vi "Day7Part2.vi"(11 "Input":string="190: 10 19\n3267: 81 40 27\n83: 17 5\n156: 15 6\n7290: 6 8 6 15\n161011: 16 10 13\n192: 17 8 14\n21037: 9 7 18 13\n292: 11 6 16 20") -> (3 "Result":u64)   [LabVIEW 2024]
uses:
  <vilib>/Utility/error.llb/Trim Whitespace One-Sided.vi
  <userlib>/_OpenG.lib/string/string.llb/openg_string.lvlib
panel:
  out "Answers":u64[](array[numeric])
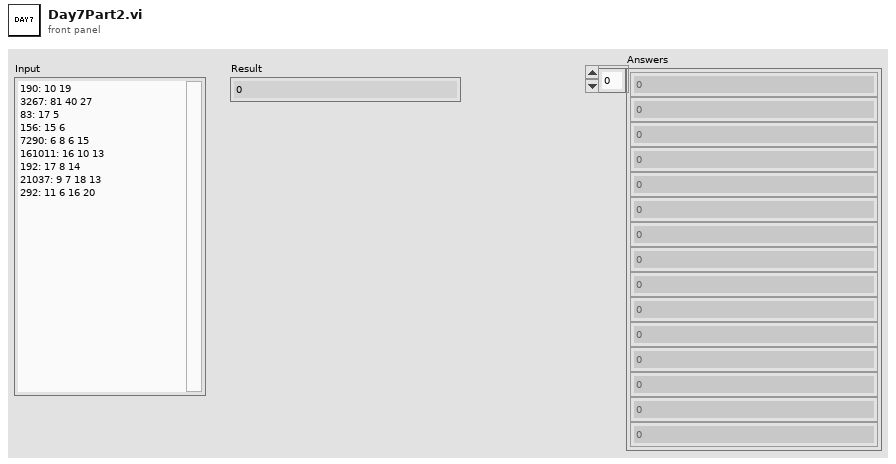
[diagram p1: front panel]
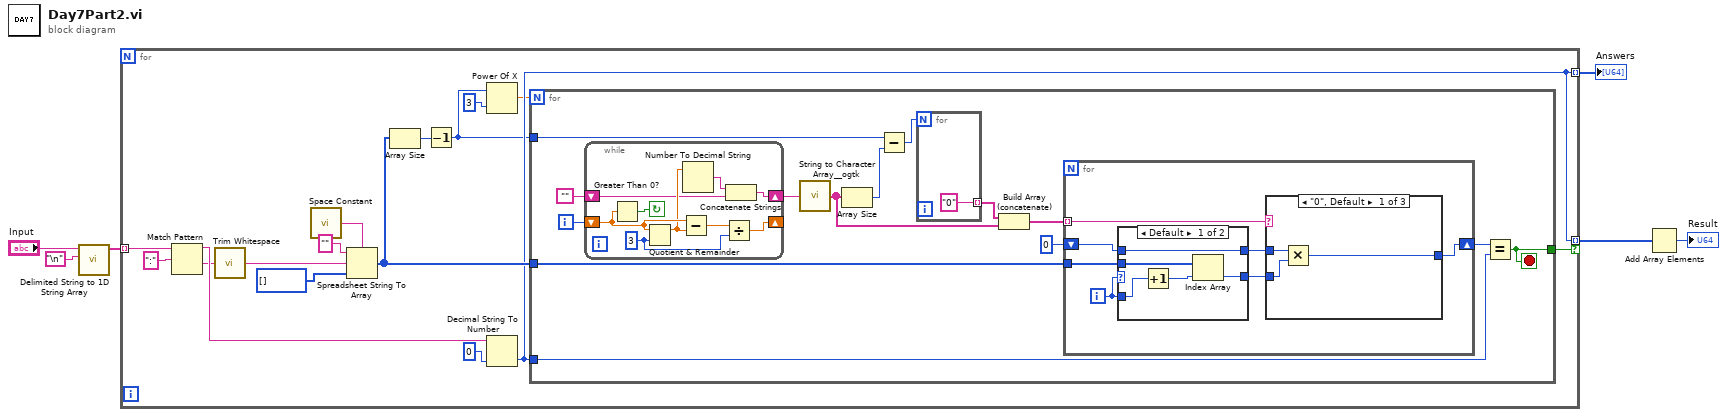
[diagram p0: block diagram]
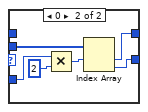
[diagram p2: hidden frame]
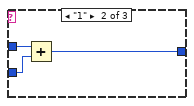
[diagram p3: hidden frame]
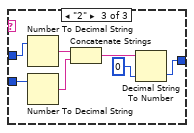
[diagram p4: hidden frame]
diagram:
  n1 = call <vilib>:"Delimited String to 1D String Array.vi"("delimiter"="\n", "delimited string"="Input") -> ("string array"=w4:string[])  [unwired: 9 in]
  n2 = for {
    tunnel: w4 -> [w22] mode=indexing
    tunnel: [w11] -> w3 mode=indexing
    tunnel: [w11] -> w2 mode=indexing if=w7
    n3 = Match Pattern(string=w22, regular expression=":") -> (before substring=w20:string, after substring=w19:string)  [unwired: 1 in, 2 out]
    n4 = call <vilib>:"Trim Whitespace.vi"("string"=w19) -> ("trimmed string"=w18:string)  [unwired: 1 in]
    n5 = call <vilib>:"Space Constant.vi"() -> ("String"=w16:string)
    n6 = Spreadsheet String To Array(delimiter (Tab)=w16, format string="", spreadsheet string=w18, array type (2D Dbl)=u64[] []) -> (array=w13:u64[])
    n7 = Array Size(array=w13) -> (size(s)=w10:i32)
    n8 = Decrement(x=w10) -> (x-1=w9:i32)
    n9 = Power Of X(1:3 ("y"), 2:w9) -> (0:w8:dbl)
    n10 = Decimal String To Number(string=w20, default (0L)=u64 0 ("default (0 I32)")) -> (number=w11:u64)  [unwired: 1 in, 1 out]
    n11 = for {
      N: w8 -> [_]
      tunnel: w13 -> [w36]
      tunnel: w11 -> [w31]
      tunnel: [w23] -> w7
      tunnel: w9 -> [w28]
      i -> [w32]
      stop <- w23 stop-if-true
      n12 = while {
        shift-right: [w46] -> w30
        shift-left: "" -> [w38]
        shift-right: [w41] -> _
        shift-left: w32 -> [w44]
        stop <- w45 continue-if-true
        w42 = 3 ("y")
        n13 = Greater Than 0?(x=w44) -> (x > 0?=w45:bool)
        n14 = Quotient & Remainder(x=w44, y=w42) -> (x-y*floor(x/y)=w40:dbl)  [unwired: 1 out]
        n15 = Subtract(x=w44, y=w40) -> (x-y=w43:dbl)
        n16 = Number To Decimal String(number=w40) -> (decimal integer string=w39:string)  [unwired: 1 in]
        n17 = Divide(x=w43, y=w42) -> (x/y=w41:dbl)
        n18 = Concatenate Strings(w39, w38) -> (w46:string)
      }
      n19 = call <userlib>:"String to Character Array__ogtk.vi"("Input String"=w30) -> ("Character Array"=w25:string[])
      n20 = Array Size(array=w25) -> (size(s)=w29:i32)
      n21 = Subtract(x=w28, y=w29) -> (x-y=w27:i32)
      n22 = for {
        N: w27 -> [_]
        tunnel: ["0"] -> w26 mode=indexing
      }
      n23 = Build Array (concatenate)(w26, w25) -> (w24:string[])
      n24 = for {
        tunnel: w36 -> [w53]
        shift-right: [w50] -> w34
        shift-left: u64 0 -> [w49]
        tunnel: w24 -> [w47] mode=indexing
        i -> [w48]
        n25 = case shown="Default" w48 {
          tunnel: w53 -> [w58 w64]
          tunnel: [w56 w63] -> w52
          tunnel: [w57 w62] -> w51
          tunnel: w49 -> [w56 _]
          tunnel: w48 -> [w55 w60]
          frame Default {
            n26 = Increment(x=w55) -> (x+1=w54:i32)
            n27 = Index Array(array=w58, index=w54) -> (element=w57:u64)
          }
          frame 0 {
            n28 = Multiply(x=w60, y=2) -> (x*y=w59:i32)
            n29 = Index Array(array=w64, index #1=w59) -> (element #1=w63:u64, element #2=w62:u64)  [unwired: 1 in]
          }
        }
        n30 = case shown="\"0\", Default" w47 {
          tunnel: w52 -> [w67 w69 w77]
          tunnel: w51 -> [w66 w70 w76]
          tunnel: [w65 w68 w71] -> w50
          frame "0", Default {
            n31 = Multiply(x=w67, y=w66) -> (x*y=w65:u64)
          }
          frame "1" {
            n32 = Add(x=w69, y=w70) -> (x+y=w68:u64)
          }
          frame "2" {
            n33 = Number To Decimal String(number=w77) -> (decimal integer string=w75:string)  [unwired: 1 in]
            n34 = Number To Decimal String(number=w76) -> (decimal integer string=w74:string)  [unwired: 1 in]
            n35 = Concatenate Strings(w75, w74) -> (w73:string)
            n36 = Decimal String To Number(string=w73, default (0L)=u64 0 ("default (0 I32)")) -> (number=w71:u64)  [unwired: 1 in, 1 out]
          }
        }
      }
      n37 = Equal?(x=w34, y=w31) -> (x = y?=w23:bool)
    }
  }
  "Answers" <- w3
  n38 = Add Array Elements(numeric array=w2) -> (sum=→"Result":u64)
